vi "Drive.vi"(8 "Drive R":dbl, 10 "Drive L":dbl) -> ()   [LabVIEW 2018]
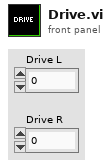
[diagram p1: front panel]
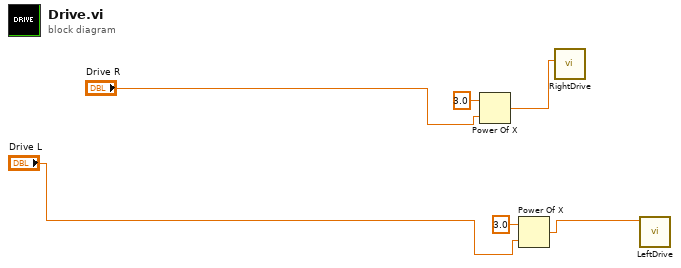
[diagram p0: block diagram]
diagram:
  n1 = Power Of X(1:"Drive R", 2:3.0 ("y")) -> (0:w3:dbl)
  n2 = Power Of X(1:"Drive L", 2:3.0 ("y")) -> (0:w1:dbl)
  n3 = call "RightDrive.vi"("Effort"=w3) -> ()  [unwired: 11 in]
  n4 = call "LeftDrive.vi"("Effort"=w1) -> ()  [unwired: 11 in]
